vi "Read type.vi"(8 "error in (no error)":errorcluster, 11 "file attributes in":refnum<class "File Attributes.lvclass">) -> (0 "error out":errorcluster, 2 "File Type":T1, 3 "file attributes out":refnum<class "File Attributes.lvclass">)   [LabVIEW 2020, in "NI_SFTP.lvlib" / "File Attributes.lvclass"]
uses:
  <vilib>/net/SFTP/File Attributes/File Attributes.lvclass
  <vilib>/net/SFTP/File Attributes/File Type.ctl
  <vilib>/net/SFTP/File Attributes/File Attributes.lvclass/File Attributes.ctl
  <vilib>/Utility/error.llb/Error Cluster From Error Code.vi
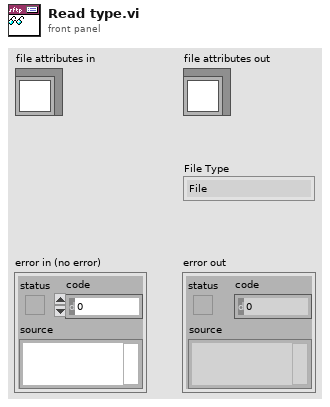
[diagram p1: front panel]
types:
  T1 = typedef "NI_SFTP.lvlib/File Attributes.lvclass/File Type.ctl" = enum16{"File", "Directory", "Character device", "Block device", "Symbolic link", "Socket", "FIFO", "Unknown"}
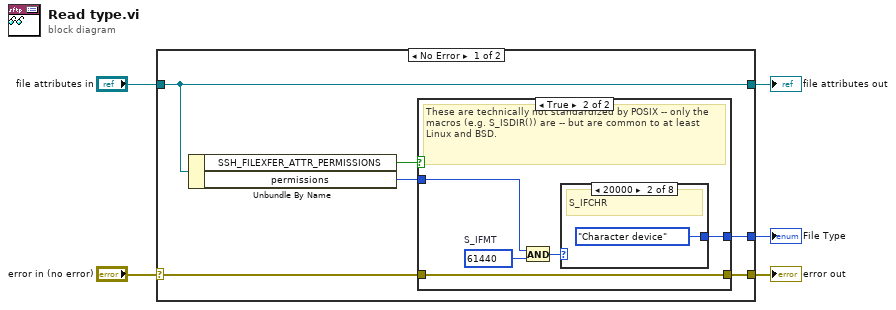
[diagram p0: block diagram]
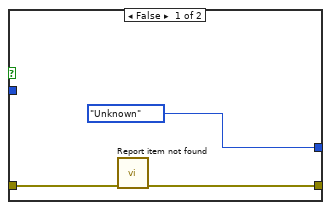
[diagram p2: hidden frame]
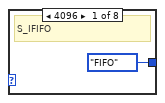
[diagram p3: hidden frame]
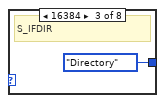
[diagram p4: hidden frame]
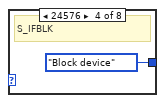
[diagram p5: hidden frame]
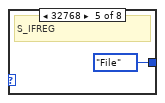
[diagram p6: hidden frame]
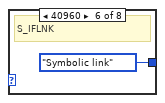
[diagram p7: hidden frame]
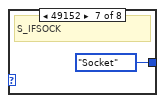
[diagram p8: hidden frame]
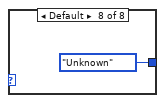
[diagram p9: hidden frame]
diagram:
  n1 = case shown="No Error" "error in (no error)" {
    selector: "error in (no error)" -> [w6 w28]
    tunnel: [w7 w28] -> w4
    tunnel: [w10 w29] -> w2
    tunnel: "file attributes in" -> [w10 w29]
    tunnel: [w9 _] -> w1
    frame No Error {
      n2 = Unbundle By Name(w10) -> ("SSH_FILEXFER_ATTR_PERMISSIONS"=w8:bool, "permissions"=w11:u32)
      n3 = case shown="True" w8 {
        tunnel: w11 -> [_ w19]
        tunnel: [File_Type."Unknown" ("File Type") w16] -> w9
        tunnel: [w13 w15] -> w7
        tunnel: w6 -> [w14 w15]
        frame False {
          n4 = call <vilib>:"Report item not found.vi"("error in (no error)"=w14) -> ("error out"=w13:errorcluster)  [unwired: 10 in]
        }
        frame True {
          w18 = u32 61440  # S_IFMT
          # "These are technically not standardized by POSIX -- only the macros (e.g. S_ISDIR()) are -- but are common to at least Linux and BSD."
          n5 = And(x=w19, y=w18) -> (x .and. y?=w17:u32)
          n6 = case shown="20000" w17 {
            tunnel: [File_Type."FIFO" ("File Type") File_Type."Character device" ("File Type") File_Type."Directory" ("File Type") File_Type."Block device" ("File Type") File_Type."File" ("File Type") File_Type."Symbolic link" ("File Type") File_Type."Socket" ("File Type") File_Type."Unknown" ("File Type")] -> w16
            frame 4096 {
              # "S_IFIFO"
            }
            frame 8192 {
              # "S_IFCHR"
            }
            frame 16384 {
              # "S_IFDIR"
            }
            frame 24576 {
              # "S_IFBLK"
            }
            frame 32768 {
              # "S_IFREG"
            }
            frame 40960 {
              # "S_IFLNK"
            }
            frame 49152 {
              # "S_IFSOCK"
            }
            frame Default {
            }
          }
        }
      }
    }
    frame Error {
    }
  }
  "error out" <- w4
  "file attributes out" <- w2
  "File Type" <- w1
